vi "VISA IO GUI.vi"(7 "write buffer":string, 8 "error in (no error)":errorcluster, 11 "VISA resource name":refnum<visa-resource-name>="TCPIP0::localhost::hislip1::INSTR") -> (0 "error out":errorcluster, 3 "read buffer":string)   [LabVIEW 2020]
doc: "abce"
panel:
  in  "Write":bool caption="Query"
  in  "Query":bool
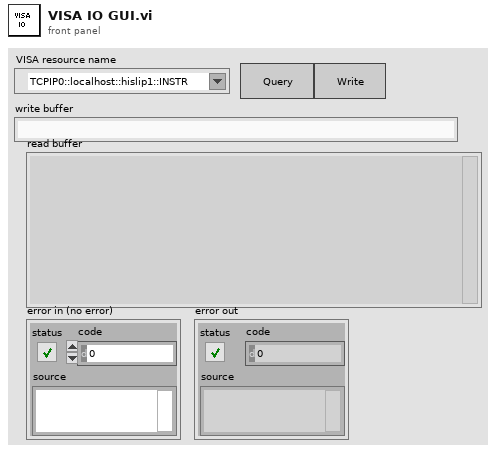
[diagram p1: front panel]
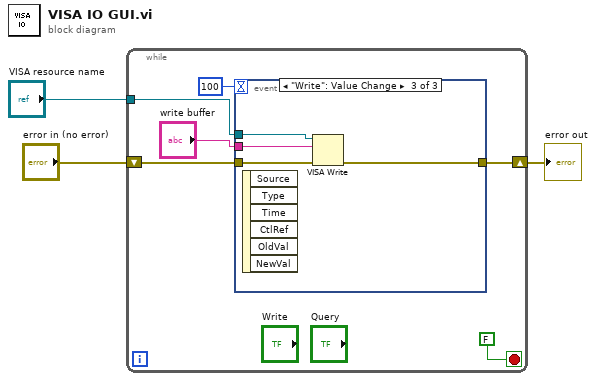
[diagram p0: block diagram]
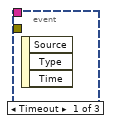
[diagram p2: hidden frame]
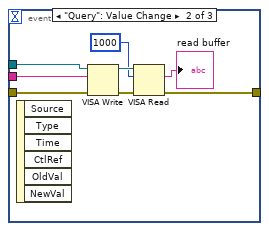
[diagram p3: hidden frame]
diagram:
  n1 = while {
    shift-right: [w8] -> w3
    shift-left: "error in (no error)" -> [w9]
    tunnel: "VISA resource name" -> [w7]
    stop <- FALSE stop-if-true
    n2 = event shown="[2] \"Write\": Value Change" {
      selector: _ -> [_ _ _]
      dyn-events: _ -> [_ _ _]
      timeout: 100 -> [_ _ _]
      tunnel: w9 -> [_ w14 w21]
      tunnel: "write buffer" -> [_ w13 w18]
      tunnel: w7 -> [_ w12 w19]
      tunnel: [_ w11 w20] -> w8
      event Timeout {
        n3 = event-data() -> ()  [unwired: 1 in, 3 out]
      }
      event "Query": Value Change {
        n4 = event-data() -> ()  [unwired: 1 in, 6 out]
        n5 = VISA Write(VISA resource name=w12, write buffer=w13, error in (no error)=w14) -> (VISA resource name out=w16:refnum<visa-resource-name>, error out=w17:errorcluster)  [unwired: 1 out]
        n6 = VISA Read(VISA resource name=w16, byte count=u32 1000, error in (no error)=w17) -> (read buffer=→"read buffer":string, error out=w11:errorcluster)  [unwired: 2 out]
      }
      event "Write": Value Change {
        n7 = event-data() -> ()  [unwired: 1 in, 6 out]
        n8 = VISA Write(VISA resource name=w19, write buffer=w18, error in (no error)=w21) -> (error out=w20:errorcluster)  [unwired: 2 out]
      }
    }
  }
  "error out" <- w3
